vi "testSpecialChar(Case13072).vi"() -> ()   [LabVIEW 2013, in "EasyXML_XML_Subset_Source_Tests.lvclass"]
uses:
  EasyXML_XML_Subset_Source_Tests.lvclass
  <vilib>/addons/_JKI Toolkits/VI Tester/TestCase.llb/TestCase.lvclass
panel:
  out "error out":errorcluster
  in  "error in (no error)":errorcluster
  out "EasyXML_XML_Subset_Source_Tests.lvclass":refnum<class "EasyXML_XML_Subset_Source_Tests.lvclass">
  in  "EasyXML_XML_Subset_Source_Tests.lvclass":refnum<class "EasyXML_XML_Subset_Source_Tests.lvclass">
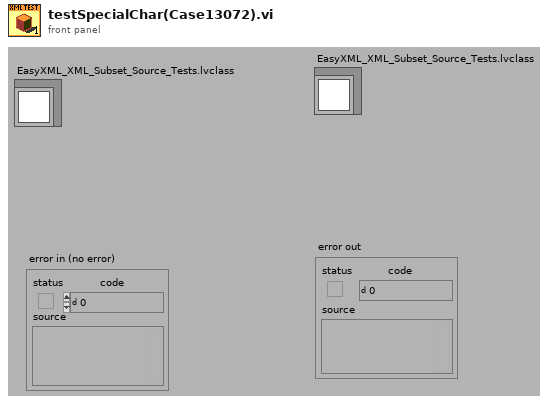
[diagram p1: front panel]
types:
  T1 = cluster{"#attributes":cluster{"name":string}, "Name":string, "Type":enum16{"none", "_Settings", "_Binder-MK-240", "_Calibration", "_Check-Equipment", "_Check-Gain-Steps_passive", "_Compare-Frequenzy-Sweeps", "_Feed-Foreward-Control", "_Frequency-Sweep", "_Get-Serialnumbers-from-User", "_Intermodulation", "_Intermodulation-Sweep", "_Noisefloor", "_Passive-Intermodulation", "_Read-Power_(Hameg-PM-8115-2)", "_Read-Value_(Fluke-45-DMM)", "_Sensitivity", "_Set-RS-485-Commando", "_Switchbox", "_User-Instruction", "amp30_Check-Coupler", "cmu_Set-Check-RX-Alarms", "cmu_Set-Check-Module-Info", "cmu_Sweep-CAL-TX-RX", "fe_Check-10MHz-Ref", "fe_Check-Cable-Monitor-Range", "fe_DAC-Voltage", "fe_Read-Cable-Monitor-Pilottone", "fe_UL-DL-Calibration(Pll)(Det)", "fft_Power-Wait-Alarm", "pa-2-98-20_Calibrate-PA", "pa-2-98-20_Read-Temp", "ppk_Sweep-Gain-Steps", "rs-485_Read-Temperature", "rs-485_Read-Version", "rs-485_Write-ID", "ru_Adjust-Gain-Range", "ru_ALS-Calibrate-PTD", "ru_ALS-Read-PTG", "ru_Calibrate-Power-Detector", "ru_Calibrate-Reflection-Detector", "ru_Check-ALC", "ru_Check-Limiter", "ru_Check-Power-Supply", "ru_Check-Temperature-Alarm", "ru_CM-Calibrate-RX", "ru_CM-Check-Function", "ru_CM-Read-TX", "ru_CMU-Set-Parameters", "ru_Config-MC", "ru_Fan-Test", "ru_Hold-Data-Check", "ru_Read-Status", "ru_Read-Temp", "ru_Read-Versions", "ru_Set/Check-Power-Alarm", "ru_SNMP-Command", "trx_adjust-check_Squelch"}, "Param":cluster{"ID":string, "Value":string}[]}
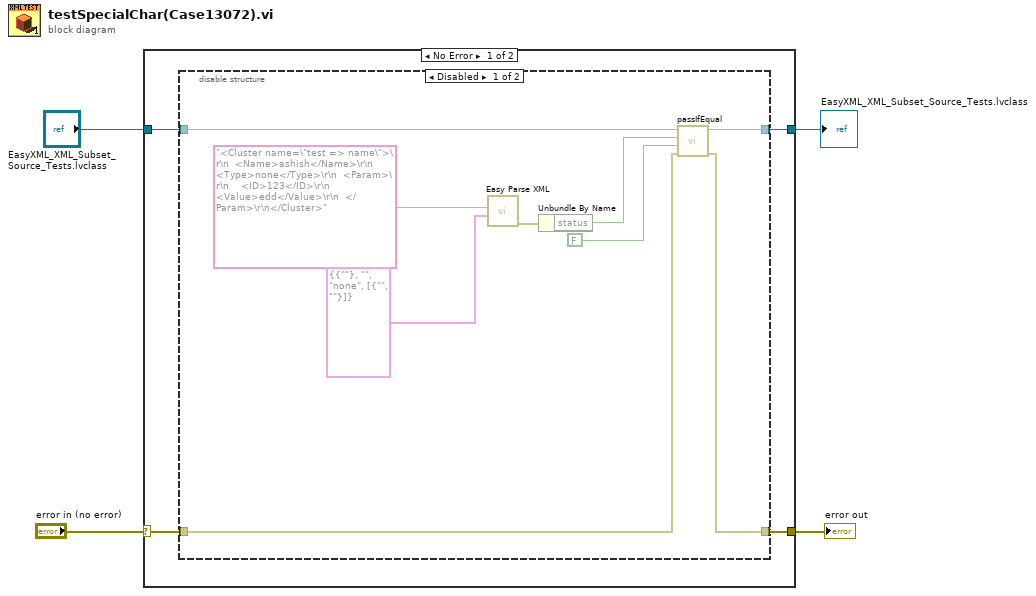
[diagram p0: block diagram]
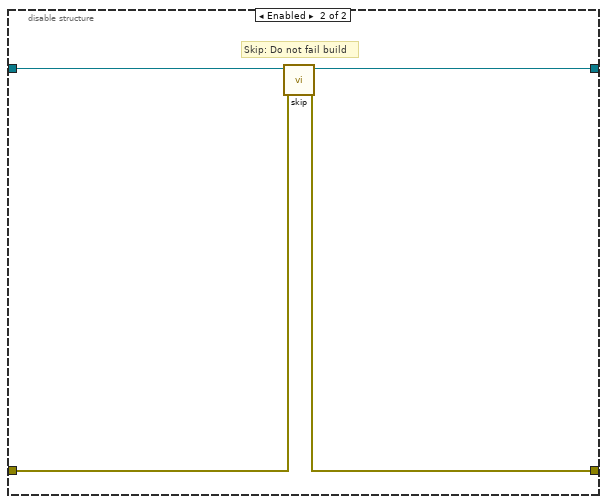
[diagram p2: hidden frame]
diagram:
  n1 = case shown="No Error" "error in (no error)" {
    selector: "error in (no error)" -> [w6 w23]
    tunnel: [w5 w23] -> w3
    tunnel: "EasyXML_XML_Subset_Source_Tests.lvclass" -> [w8 w22]
    tunnel: [w7 w22] -> w1
    frame No Error {
      n2 = disable-structure shown="Disabled" {
        disable-tunnel: w8 -> [w17 w21]
        disable-tunnel: [w16 w18] -> w7
        disable-tunnel: w6 -> [w10 w20]
        disable-tunnel: [w9 w19] -> w5
        frame Disabled {
          n3 = call "Easy Parse XML.vi"("LabVIEW Data (Type)"=T1 {"#attributes"={"name"=""}, "Name"="", "Type"=enum."none", "Param"=[{"ID"="", "Value"=""}]} ("Cluster"), "XML String"="<Cluster name=\"test => name\">\r\n  <Name>ashish</Name>\r\n  <Type>none</Type>\r\n  <Param>\r\n    <ID>123</ID>\r\n    <Value>edd</Value>\r\n  </Param>\r\n</Cluster>") -> ("error out"=w13:errorcluster)  [unwired: 8 in, 1 out]
          n4 = Unbundle By Name(w13) -> ("status"=w12:bool)
          n5 = call-dynamic "passIfEqual.vi"("error in (no error)"=w10, "y"=FALSE ("status"), "x"=w12, "TestCase in"=w17) -> ("error out"=w9:errorcluster, "TestCase out"=w16:refnum<class "EasyXML_XML_Subset_Source_Tests.lvclass">)  [unwired: 6 in]
        }
        frame Enabled {
          # "Skip: Do not fail build"
          n6 = call <vilib>:"skip.vi"("error in (no error)"=w20, "TestCase in"=w21) -> ("error out"=w19:errorcluster, "TestCase out"=w18:refnum<class "EasyXML_XML_Subset_Source_Tests.lvclass">)  [unwired: 8 in]
        }
      }
    }
    frame Error {
    }
  }
  "EasyXML_XML_Subset_Source_Tests.lvclass" <- w1
  "error out" <- w3
